vi "BK-5492C_Main.vi"(6 "Open/Close?":bool=TRUE, 8 "error in":errorcluster, 10 "Parameters":string, 11 "VISA resource name":refnum<visa-resource-name>="USB0::0x3121::0x5000::556K20102::INSTR") -> (0 "error out":errorcluster, 2 "Measurement Function":i32, 3 "Result Value":dbl)   [LabVIEW 2018]
panel:
  out "Measurement":dbl
  # "DMM BK-5492C"
  # "PARAMETERS"
  # "V-DC>0              --Auto Range"
  # "V-DC>0,1          --Manual Range (0,1 1 10 100 1000)"
  # "V-AC>0            --Auto Range"
  # "V-AC>100         --Manual Range (0,1 1 10 100 700)"
  # "R-2W>0              --Auto Range"
  # "R-2W>0,1          --Manual Range (10 100 1K 100K 1M 10M 100M)"
  # "R-4W>0              --Auto Range"
  # "R-2W>0,1          --Manual Range (10 100 1K 100K 1M 10M 100M)"
  # "C>0                   --Auto Range"
  # "C>10nF              --Manual Range (1nF 10nF 100nF 1uF 100uF 1mF 10mF)"
  # "D                       --Auto Range  (Diode)"
  # "F>0                    --Auto (Volt) Range  measure->(Frequency Hz)"
  # "F>100         -        -Manual (Volt)Range (0,1 1 10 100 700)"
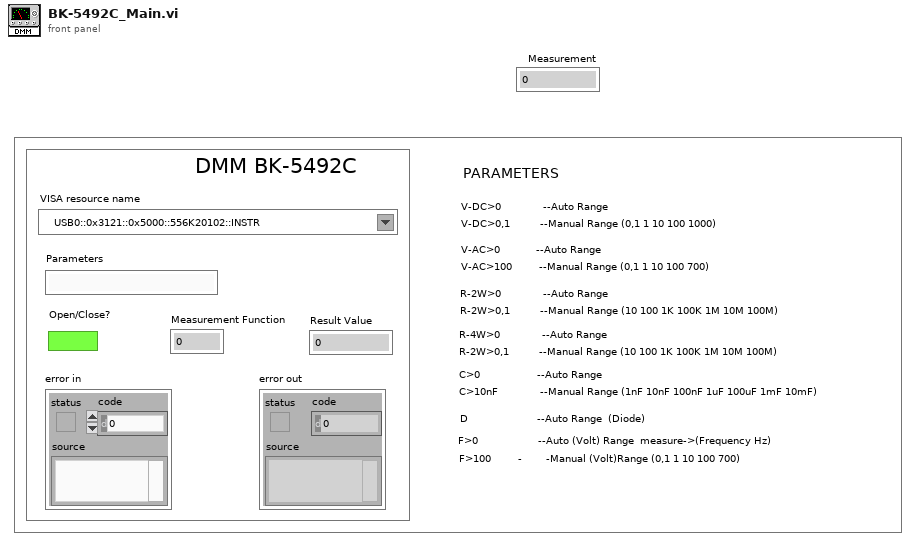
[diagram p1: front panel]
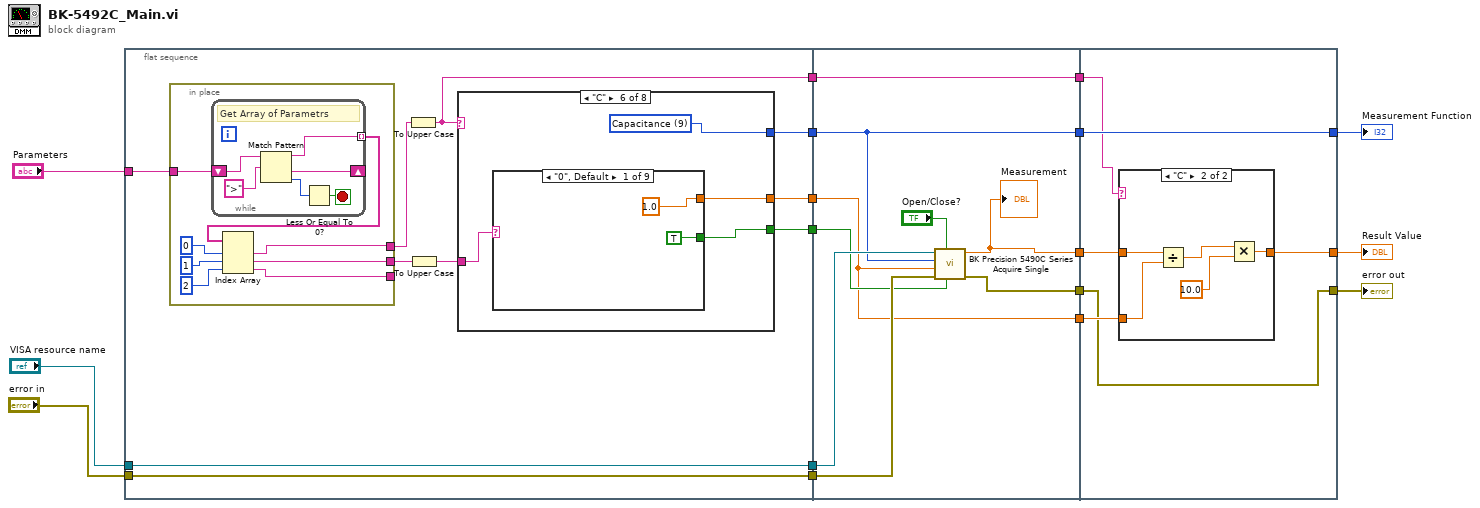
[diagram p0: block diagram]
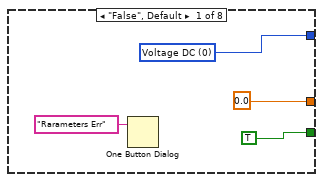
[diagram p2: hidden frame]
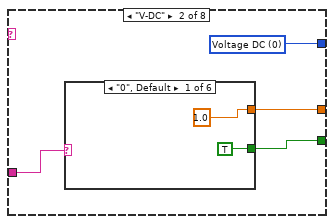
[diagram p3: hidden frame]
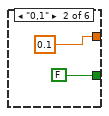
[diagram p4: hidden frame]
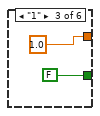
[diagram p5: hidden frame]
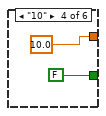
[diagram p6: hidden frame]
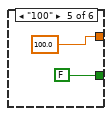
[diagram p7: hidden frame]
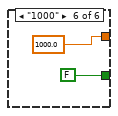
[diagram p8: hidden frame]
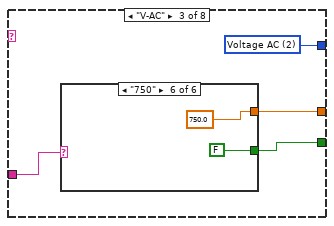
[diagram p9: hidden frame]
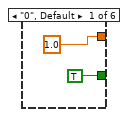
[diagram p10: hidden frame]
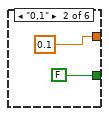
[diagram p11: hidden frame]
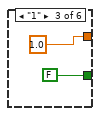
[diagram p12: hidden frame]
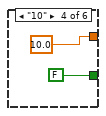
[diagram p13: hidden frame]
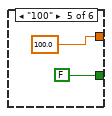
[diagram p14: hidden frame]
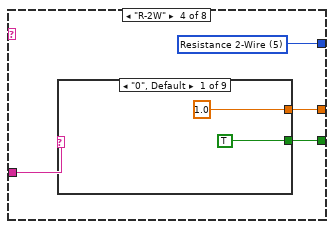
[diagram p15: hidden frame]
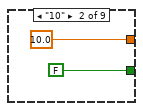
[diagram p16: hidden frame]
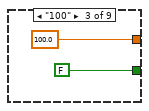
[diagram p17: hidden frame]
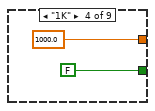
[diagram p18: hidden frame]
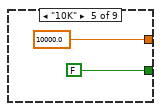
[diagram p19: hidden frame]
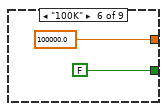
[diagram p20: hidden frame]
diagram:
  n1 = flat-sequence {
    tunnel: "Parameters" -> [w27]
    tunnel: "error in" -> [w26]
    tunnel: [w26] -> w16
    tunnel: [w25] -> w12
    tunnel: "VISA resource name" -> [w25]
    tunnel: [w24] -> w10
    tunnel: [w23] -> w9
    tunnel: [w22] -> w8
    tunnel: [w18] -> w1
    tunnel: w16 -> [w171]
    tunnel: w12 -> [w168]
    tunnel: w10 -> [w167]
    tunnel: w9 -> [w163]
    tunnel: w8 -> [w166]
    tunnel: [w170] -> w6
    tunnel: [w169] -> w5
    tunnel: [w166] -> w4
    tunnel: [w163] -> w3
    tunnel: [w164] -> w2
    tunnel: w1 -> [w164]
    tunnel: [w177] -> w7
    tunnel: [w176] -> w13
    tunnel: [w172] -> w14
    tunnel: w6 -> [w172]
    tunnel: w5 -> [w175]
    tunnel: w4 -> [w177]
    tunnel: w3 -> [w174]
    tunnel: w2 -> [w173]
    frame #0 {
      n2 = in-place {
        in-place-border: w27 -> [w153]
        in-place-border: [w151] -> w19
        in-place-border: [w150] -> w20
        in-place-border: [w149] -> _
        n3 = while {
          shift-right: [w160] -> _
          shift-left: w153 -> [w161]
          tunnel: [w157] -> w152 mode=indexing
          stop <- w159 stop-if-true
          # "Get Array of Parametrs"
          n4 = Match Pattern(string=w161, regular expression=">") -> (before substring=w157:string, after substring=w160:string, offset past match=w158:i32)  [unwired: 1 in, 1 out]
          n5 = Less Or Equal To 0?(x=w158) -> (x <= 0?=w159:bool)
        }
        n6 = Index Array(array=w152, index #1=0 ("index"), index #2=1 ("index"), index #3=2 ("index")) -> (element #1=w151:string, element #2=w150:string, element #3=w149:string)
      }
      n7 = To Upper Case(1:w19) -> (0:w18:string)
      n8 = To Upper Case(1:w20) -> (0:w21:string)
      n9 = case shown="\"C\"" w18 {
        tunnel: [w30 w32 w51 w67 w89 w111 w132 w136] -> w22
        tunnel: w21 -> [_ w35 w48 w64 w88 w110 _ w133]
        tunnel: [TRUE w34 w50 w66 w87 w109 FALSE ("Auto Range (T: Enable)") w134] -> w24
        tunnel: [0.0 w33 w49 w65 w86 w108 0.0 ("Manual Range (1)") w135] -> w23
        frame "False", Default {
          w30 = 0 items=["Voltage DC", "Voltage DC Ratio", "Voltage AC", "Current DC", "Current AC", "Resistance 2-Wire", "Resistance 4-Wire", "Frequency", "Period", "Capacitance", "Continuity", "Diode", "Temperature"] ("Measurement Function (0: Voltage DC)")
          n10 = One Button Dialog(message="Rarameters Err") -> ()  [unwired: 1 in, 1 out]
        }
        frame "V-DC" {
          w32 = 0 items=["Voltage DC", "Voltage DC Ratio", "Voltage AC", "Current DC", "Current AC", "Resistance 2-Wire", "Resistance 4-Wire", "Frequency", "Period", "Capacitance", "Continuity", "Diode", "Temperature"] ("Measurement Function (0: Voltage DC)")
          n11 = case shown="\"0\", Default" w35 {
            tunnel: [TRUE ("Auto Range (T: Enable)") FALSE ("Auto Range (T: Enable)") FALSE ("Auto Range (T: Enable)") FALSE ("Auto Range (T: Enable)") FALSE ("Auto Range (T: Enable)") FALSE ("Auto Range (T: Enable)")] -> w34
            tunnel: [1.0 ("Manual Range (1)") 0.1 ("Manual Range (1)") 1.0 ("Manual Range (1)") 10.0 ("Manual Range (1)") 100.0 ("Manual Range (1)") 1000.0 ("Manual Range (1)")] -> w33
            frame "0", Default {
            }
            frame "0,1" {
            }
            frame "1" {
            }
            frame "10" {
            }
            frame "100" {
            }
            frame "1000" {
            }
          }
        }
        frame "V-AC" {
          w51 = 2 items=["Voltage DC", "Voltage DC Ratio", "Voltage AC", "Current DC", "Current AC", "Resistance 2-Wire", "Resistance 4-Wire", "Frequency", "Period", "Capacitance", "Continuity", "Diode", "Temperature"] ("Measurement Function (0: Voltage DC)")
          n12 = case shown="\"750\"" w48 {
            tunnel: [TRUE ("Auto Range (T: Enable)") FALSE ("Auto Range (T: Enable)") FALSE ("Auto Range (T: Enable)") FALSE ("Auto Range (T: Enable)") FALSE ("Auto Range (T: Enable)") FALSE ("Auto Range (T: Enable)")] -> w50
            tunnel: [1.0 ("Manual Range (1)") 0.1 ("Manual Range (1)") 1.0 ("Manual Range (1)") 10.0 ("Manual Range (1)") 100.0 ("Manual Range (1)") 750.0 ("Manual Range (1)")] -> w49
            frame "0", Default {
            }
            frame "0,1" {
            }
            frame "1" {
            }
            frame "10" {
            }
            frame "100" {
            }
            frame "750" {
            }
          }
        }
        frame "R-2W" {
          w67 = 5 items=["Voltage DC", "Voltage DC Ratio", "Voltage AC", "Current DC", "Current AC", "Resistance 2-Wire", "Resistance 4-Wire", "Frequency", "Period", "Capacitance", "Continuity", "Diode", "Temperature"] ("Measurement Function (0: Voltage DC)")
          n13 = case shown="\"0\", Default" w64 {
            tunnel: [TRUE ("Auto Range (T: Enable)") FALSE ("Auto Range (T: Enable)") FALSE ("Auto Range (T: Enable)") FALSE ("Auto Range (T: Enable)") FALSE ("Auto Range (T: Enable)") FALSE ("Auto Range (T: Enable)") FALSE ("Auto Range (T: Enable)") FALSE ("Auto Range (T: Enable)") FALSE ("Auto Range (T: Enable)")] -> w66
            tunnel: [1.0 ("Manual Range (1)") 10.0 ("Manual Range (1)") 100.0 ("Manual Range (1)") 1000.0 ("Manual Range (1)") 10000.0 ("Manual Range (1)") 100000.0 ("Manual Range (1)") 1000000.0 ("Manual Range (1)") 10000000.0 ("Manual Range (1)") 100000000.0 ("Manual Range (1)")] -> w65
            frame "0", Default {
            }
            frame "10" {
            }
            frame "100" {
            }
            frame "1K" {
            }
            frame "10K" {
            }
            frame "100K" {
            }
            frame "1M" {
            }
            frame "10M" {
            }
            frame "100M" {
            }
          }
        }
        frame "R-4W" {
          w89 = 6 items=["Voltage DC", "Voltage DC Ratio", "Voltage AC", "Current DC", "Current AC", "Resistance 2-Wire", "Resistance 4-Wire", "Frequency", "Period", "Capacitance", "Continuity", "Diode", "Temperature"] ("Measurement Function (0: Voltage DC)")
          n14 = case shown="\"100M\"" w88 {
            tunnel: [TRUE ("Auto Range (T: Enable)") FALSE ("Auto Range (T: Enable)") FALSE ("Auto Range (T: Enable)") FALSE ("Auto Range (T: Enable)") FALSE ("Auto Range (T: Enable)") FALSE ("Auto Range (T: Enable)") FALSE ("Auto Range (T: Enable)") FALSE ("Auto Range (T: Enable)") FALSE ("Auto Range (T: Enable)")] -> w87
            tunnel: [1.0 ("Manual Range (1)") 10.0 ("Manual Range (1)") 100.0 ("Manual Range (1)") 1000.0 ("Manual Range (1)") 10000.0 ("Manual Range (1)") 100000.0 ("Manual Range (1)") 1000000.0 ("Manual Range (1)") 10000000.0 ("Manual Range (1)") 100000000.0 ("Manual Range (1)")] -> w86
            frame "0", Default {
            }
            frame "10" {
            }
            frame "100" {
            }
            frame "1K" {
            }
            frame "10K" {
            }
            frame "100K" {
            }
            frame "1M" {
            }
            frame "10M" {
            }
            frame "100M" {
            }
          }
        }
        frame "C" {
          w111 = 9 items=["Voltage DC", "Voltage DC Ratio", "Voltage AC", "Current DC", "Current AC", "Resistance 2-Wire", "Resistance 4-Wire", "Frequency", "Period", "Capacitance", "Continuity", "Diode", "Temperature"] ("Measurement Function (0: Voltage DC)")
          n15 = case shown="\"0\", Default" w110 {
            tunnel: [TRUE ("Auto Range (T: Enable)") FALSE ("Auto Range (T: Enable)") FALSE ("Auto Range (T: Enable)") FALSE ("Auto Range (T: Enable)") FALSE ("Auto Range (T: Enable)") FALSE ("Auto Range (T: Enable)") FALSE ("Auto Range (T: Enable)") FALSE ("Auto Range (T: Enable)") FALSE ("Auto Range (T: Enable)")] -> w109
            tunnel: [1.0 ("Manual Range (1)") 1e-09 ("Manual Range (1)") 1e-08 ("Manual Range (1)") 1e-07 ("Manual Range (1)") 1e-06 ("Manual Range (1)") 1e-05 ("Manual Range (1)") 0.0001 ("Manual Range (1)") 0.001 ("Manual Range (1)") 0.01 ("Manual Range (1)")] -> w108
            frame "0", Default {
            }
            frame "1NF" {
            }
            frame "10NF" {
            }
            frame "100NF" {
            }
            frame "1UF" {
            }
            frame "10UF" {
            }
            frame "100UF" {
            }
            frame "1MF" {
              (unwired) 1000000.0
            }
            frame "10MF" {
            }
          }
        }
        frame "D" {
          w132 = 11 items=["Voltage DC", "Voltage DC Ratio", "Voltage AC", "Current DC", "Current AC", "Resistance 2-Wire", "Resistance 4-Wire", "Frequency", "Period", "Capacitance", "Continuity", "Diode", "Temperature"] ("Measurement Function (0: Voltage DC)")
        }
        frame "F" {
          w136 = 7 items=["Voltage DC", "Voltage DC Ratio", "Voltage AC", "Current DC", "Current AC", "Resistance 2-Wire", "Resistance 4-Wire", "Frequency", "Period", "Capacitance", "Continuity", "Diode", "Temperature"] ("Measurement Function (0: Voltage DC)")
          n16 = case shown="\"750\"" w133 {
            tunnel: [TRUE ("Auto Range (T: Enable)") FALSE ("Auto Range (T: Enable)") FALSE ("Auto Range (T: Enable)") FALSE ("Auto Range (T: Enable)") FALSE ("Auto Range (T: Enable)") FALSE ("Auto Range (T: Enable)")] -> w134
            tunnel: [1.0 ("Manual Range (1)") 0.1 ("Manual Range (1)") 1.0 ("Manual Range (1)") 10.0 ("Manual Range (1)") 100.0 ("Manual Range (1)") 750.0 ("Manual Range (1)")] -> w135
            frame "0", Default {
            }
            frame "0,1" {
            }
            frame "1" {
            }
            frame "10" {
            }
            frame "100" {
            }
            frame "750" {
            }
          }
        }
      }
    }
    frame #1 {
      n17 = call "BK Precision 5490C Series Acquire Single.vi"("Auto Range (T: Enable)"=w167, "Open?"="Open/Close?", "error in"=w171, "Manual Range (1)"=w163, "Measurement Function (0: Voltage DC)"=w166, "VISA resource name"=w168) -> ("error out"=w170:errorcluster, "Measurement"=w169:dbl)  [unwired: 4 in]
      "Measurement" <- w169
    }
    frame #2 {
      n18 = case shown="\"C\"" w173 {
        tunnel: [w178 w181] -> w176
        tunnel: w175 -> [w178 w183]
        tunnel: w174 -> [_ w182]
        frame "Else", Default {
        }
        frame "C" {
          n19 = Divide(x=w183, y=w182) -> (x/y=w180:dbl)
          n20 = Multiply(x=w180, y=10.0) -> (x*y=w181:dbl)
        }
      }
    }
  }
  "error out" <- w14
  "Result Value" <- w13
  "Measurement Function" <- w7
